vi "MAP_AREA.vi"() -> (0 "MAP_DIM":i16=4096)   [LabVIEW 2020]
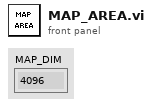
[diagram p1: front panel]
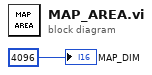
[diagram p0: block diagram]
diagram:
  "MAP_DIM" <- i16 4096
